vi "EDGE DETCTION.vi"(8 "error in (no error)":errorcluster, 10 "GAIN VALUE":dbl=0.00109 format="%#_13g", 11 "Image Path":path=path "C:/LAB-IQ 150/Images/V3_TEST_2A.jpg") -> (0 "error out":errorcluster, 2 "return value":cluster{string, string, dbl, dbl, dbl})   [LabVIEW 2025]
panel:
  out "Predicted":string
  out "String":string
  out "Comparison":string
  out "Major_Axis":dbl
  out "Minor_Axis":dbl
  out "Avg Wear Scar":dbl
  # "12823"
  # "1282335808"
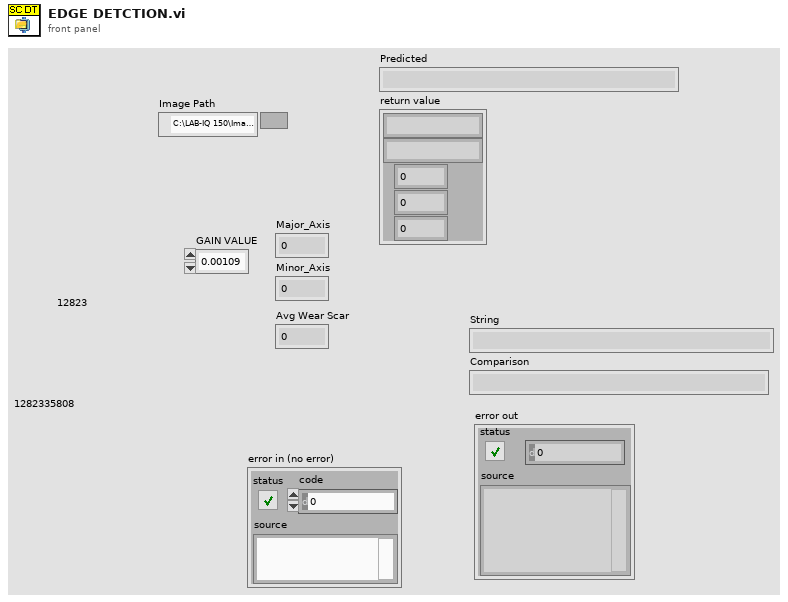
[diagram p1: front panel]
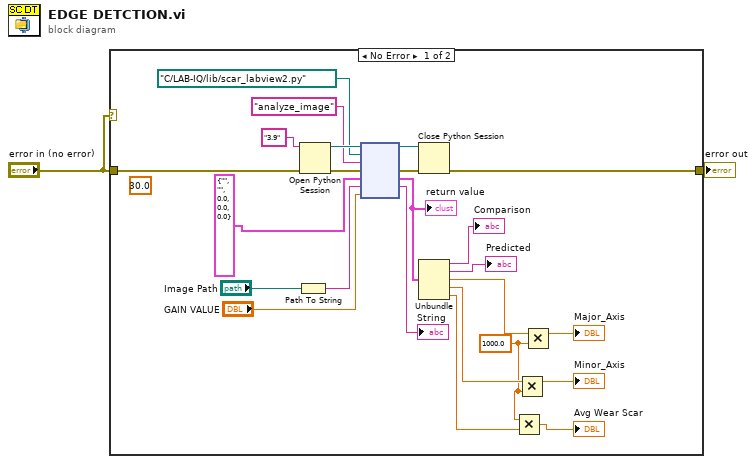
[diagram p0: block diagram]
diagram:
  n1 = case shown="No Error" "error in (no error)" {
    tunnel: "error in (no error)" -> [w13 w27]
    tunnel: [w12 w27] -> w2
    frame No Error {
      w3 = 1000.0 ("y")
      (unwired) 30.0
      n2 = Path To String(path="Image Path") -> (string=w18:string)
      n3 = Open Python Session(python version="3.9" ("Python version"), 3:w13) -> (session out=w25:refnum<k35>, error out=w22:errorcluster)  [unwired: 1 in]
      n4 = node(w25, path "C:/LAB-IQ/lib/scar_labview2.py" ("Python path"), "analyze_image" ("function name"), w22, cluster{string, string, dbl, dbl, dbl} {"", "", 0.0, 0.0, 0.0}, w18, "GAIN VALUE") -> (w23:refnum<k35>, w24:errorcluster, w15:cluster{string, string, dbl, dbl, dbl}, →"String":string)  [unwired: 1 in, 2 out]
      "return value" <- w15
      n5 = Close Python Session(session in=w23, error in=w24) -> (11:w12:errorcluster)
      n6 = Unbundle(w15) -> (→"Comparison":string, →"Predicted":string, w8:dbl, w9:dbl, w10:dbl)
      n7 = Multiply(x=w3, y=w10) -> (x*y=→"Avg Wear Scar":dbl)
      n8 = Multiply(x=w9, y=w3) -> (x*y=→"Minor_Axis":dbl)
      n9 = Multiply(x=w8, y=w3) -> (x*y=→"Major_Axis":dbl)
    }
    frame Error {
    }
  }
  "error out" <- w2
